vi "Save Layout.vi"(8 "error in (no error)":errorcluster, 10 "key":string, 11 "input cluster":T5) -> (0 "error out":errorcluster, 3 "map out":map{string, T1}(c390))   [LabVIEW 2020, in "MDI ViewManager.lvlib"]
uses:
  MDI ViewManager.lvlib
  Typedef/Layout.ctl
  <vilib>/Utility/miscctls.llb/LVPointTypeDef.ctl
  <vilib>/Utility/miscctls.llb/LVBoundsTypeDef.ctl
  <vilib>/Utility/miscctls.llb/LVPositionTypeDef.ctl
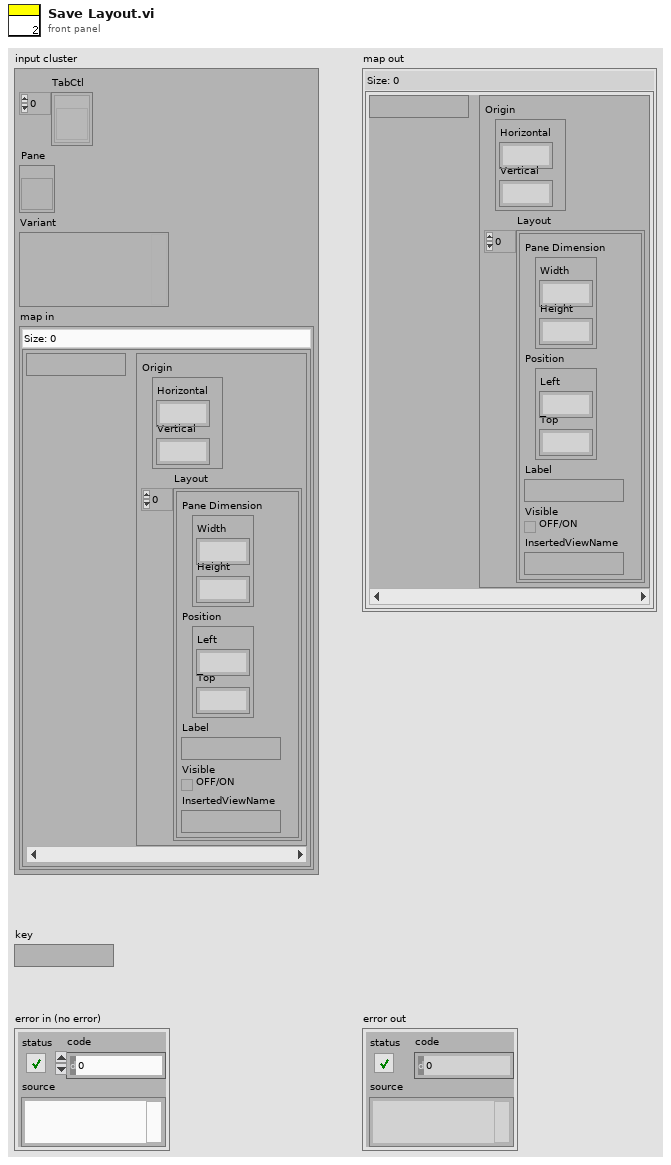
[diagram p1: front panel]
types:
  T1 = typedef "MDI ViewManager.lvlib/Layout.ctl" = cluster{"Origin":T2, "Layout":cluster{"Pane Dimension":T3, "Position":T4, "Label":string, "Visible":bool, "InsertedViewName":string}[]}
  T2 = typedef "LVPointTypeDef.ctl" = cluster{"Horizontal":i16, "Vertical":i16}
  T3 = typedef "LVBoundsTypeDef.ctl" = cluster{"Width":u32, "Height":u32}
  T4 = typedef "LVPositionTypeDef.ctl" = cluster{"Left":i32, "Top":i32}
  T5 = cluster{"TabCtl":refnum<vi>[], "Pane":refnum<vi>, "Variant":variant, "map in":map{string, T1}}
  T6 = cluster{"Pane Dimension":T3, "Position":T4, "Label":string, "Visible":bool, "InsertedViewName":string}
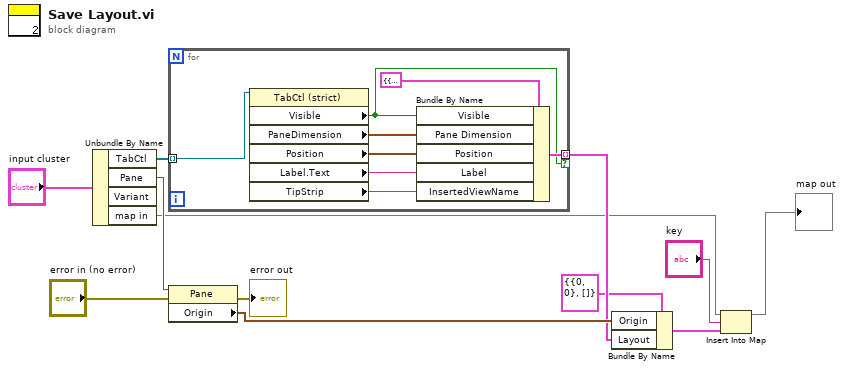
[diagram p0: block diagram]
diagram:
  n1 = Unbundle By Name("input cluster") -> ("TabCtl"=w10:refnum<vi>[], "Pane"=w9:refnum<vi>, "map in"=w5:map{string, T1})  [unwired: 1 out]
  n2 = for {
    tunnel: w10 -> [w15] mode=indexing
    tunnel: [w18] -> w11 mode=indexing if=w16
    n3 = property class="TabCtl (strict)"(reference=w15) -> ("Visible"=w16:bool, "PaneDimension"=w20:T3, "Position"=w19:T4, "Label.Text"=w14:string, "TipStrip"=w13:string)  [unwired: 1 in, 2 out]
    n4 = Bundle By Name(cluster=T6 {"Pane Dimension"={"Width"=0, "Height"=0}, "Position"={"Left"=0, "Top"=0}, "Label"="", "Visible"=FALSE, "InsertedViewName"=""}, "Visible"=w16, "Pane Dimension"=w20, "Position"=w19, "Label"=w14, "InsertedViewName"=w13) -> (w18:T6)
  }
  n5 = property class="Pane"(reference=w9, error in="error in (no error)") -> (error out=→"error out":errorcluster, "Origin"=w12:T2)  [unwired: 1 out]
  n6 = Bundle By Name(cluster=T1 {"Origin"={"Horizontal"=0, "Vertical"=0}, "Layout"=[]} ("value"), "Origin"=w12, "Layout"=w11) -> (w2:T1)
  n7 = Insert Into Map(map in=w5, key="key", value=w2) -> (map out=→"map out":map{string, T1})  [unwired: 2 out]
